vi "Plugin-002-CalibrationTest.vi"(0 "Configuration Page":refnum<class "Material-ConfigPage.lvclass">, 11 "error in":errorcluster) -> (15 "error out":errorcluster)   [LabVIEW 2014, in "Calibration-RunTest.lvclass"]
doc: "DisplayName=\"Deploy Configuration Template\"\nDescription=\"This VI serves as a template page for the Deploy Configuration UI.\""
uses:
  Plugins/Run Calibration Test/Calibration-RunTest.lvclass
  Reuse Library/featherweight/Core/Sequencer/FTW-Sequencer.lvclass
  Reuse Library/featherweight/Core/Messaging/Message.Actor/FTW-Message-Actor.lvclass
  Material-ConfigPage.lvclass
  <vilib>/Utility/miscctls.llb/LVPointTypeDef.ctl
  Plugins/Motion Control/Motion-ControlAll.lvclass
  Reuse Library/Keyence LK-G5000/Keyence LK-G5000.lvlib
  Reuse Library/Keyence LK-G5000/Public/Constant/Comm Interface.ctl
  <vilib>/Utility/error.llb/Error Cluster From Error Code.vi
  <vilib>/ErrorRing/Error Ring.xnode
panel:
  out "Thickness Measured Real Time":dbl format="%_6g"
  in  "Stop Button":bool
  out "Calibration Complete":bool
  in  "Collect Cal Data":bool
  out "Line 3 Calibration Data":dbl[](graph)
  out "Line 2 Calibration Data":dbl[](graph)
  out "Line 1 Calibration Data":dbl[](graph)
  # "Inputs"
  # "Outputs"
  # "Second Plugin"
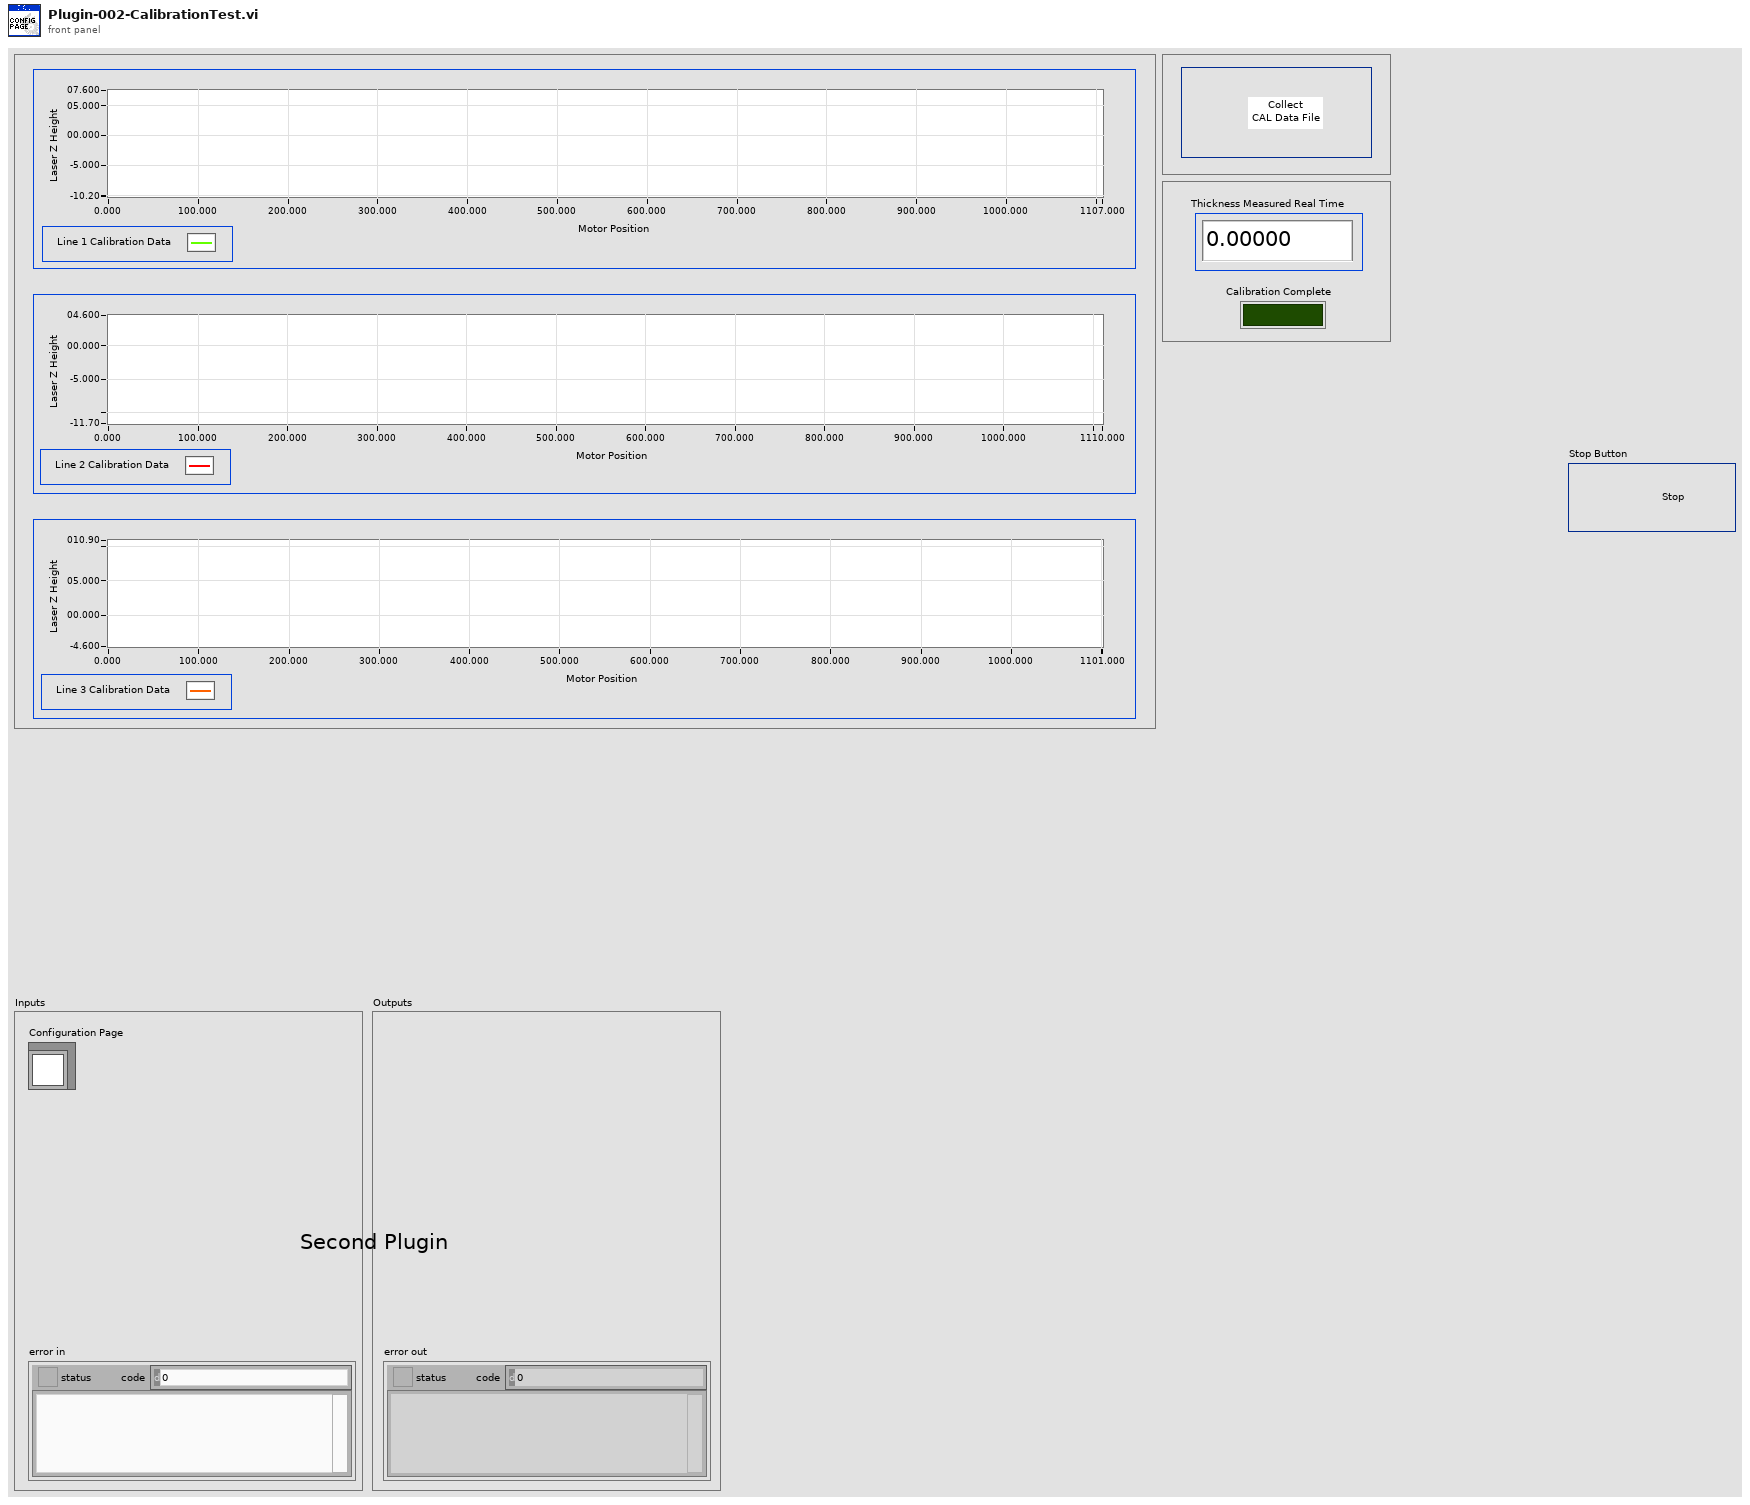
[diagram p1: front panel]
types:
  T1 = enum8{"Enabled", "Disabled", "Disabled and Grayed Out"}
  T2 = typedef "Keyence LK-G5000.lvlib/Comm Interface.ctl" = enum8{"USB", "ETHERNET"}
  T3 = typedef "LVPointTypeDef.ctl" = cluster{"Horizontal":i16, "Vertical":i16}
  T4 = cluster{"PageCommands":refnum<event-registration>}
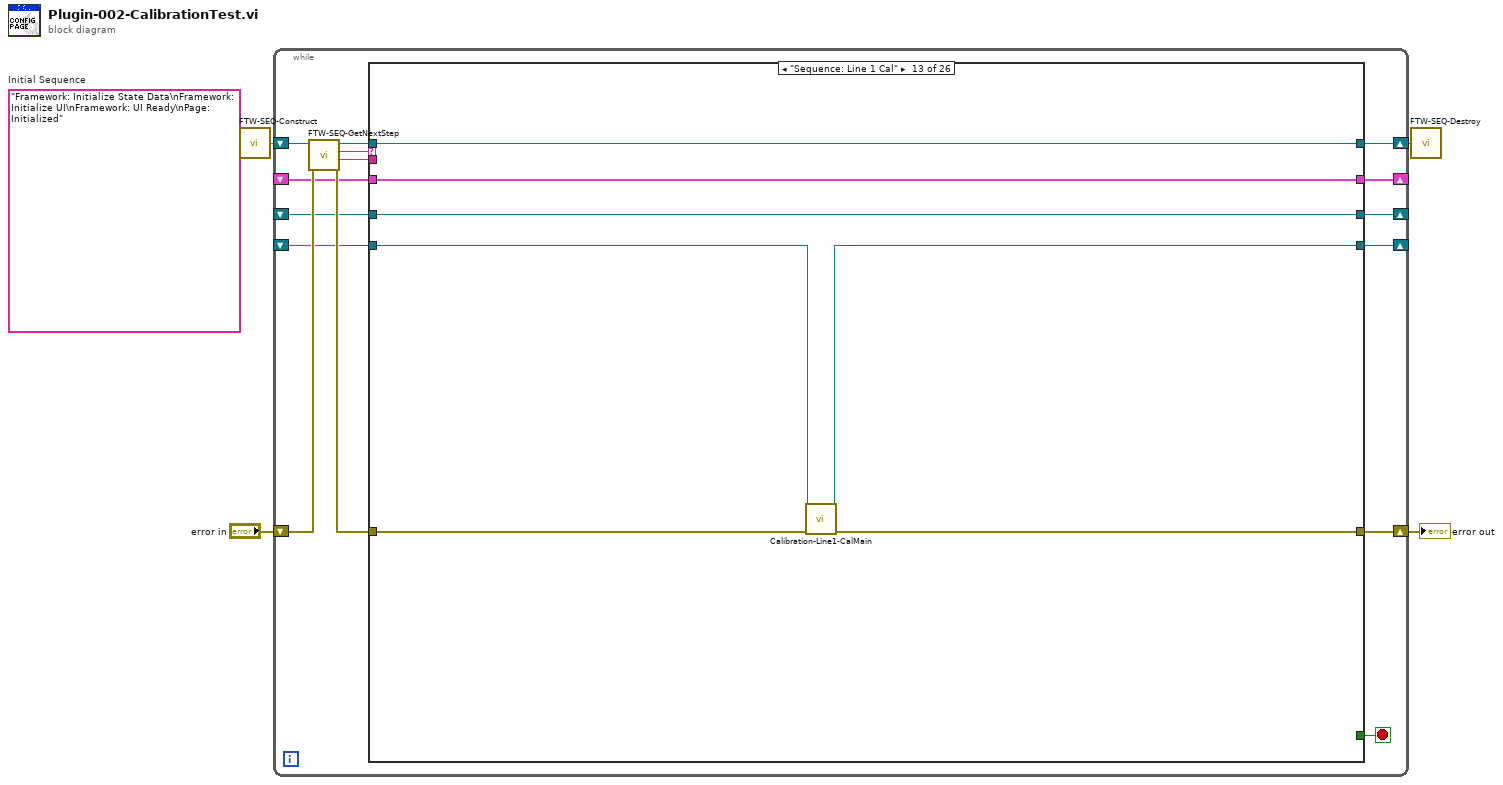
[diagram p0: block diagram]
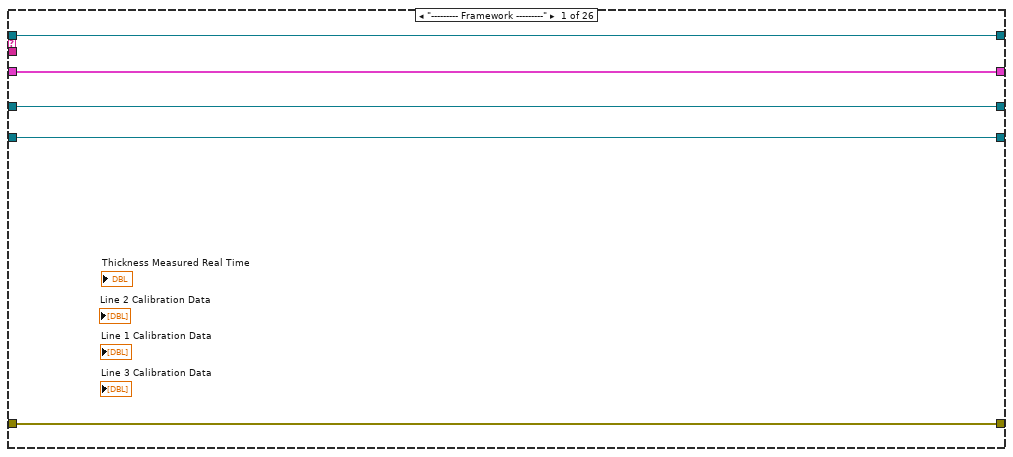
[diagram p2: hidden frame]
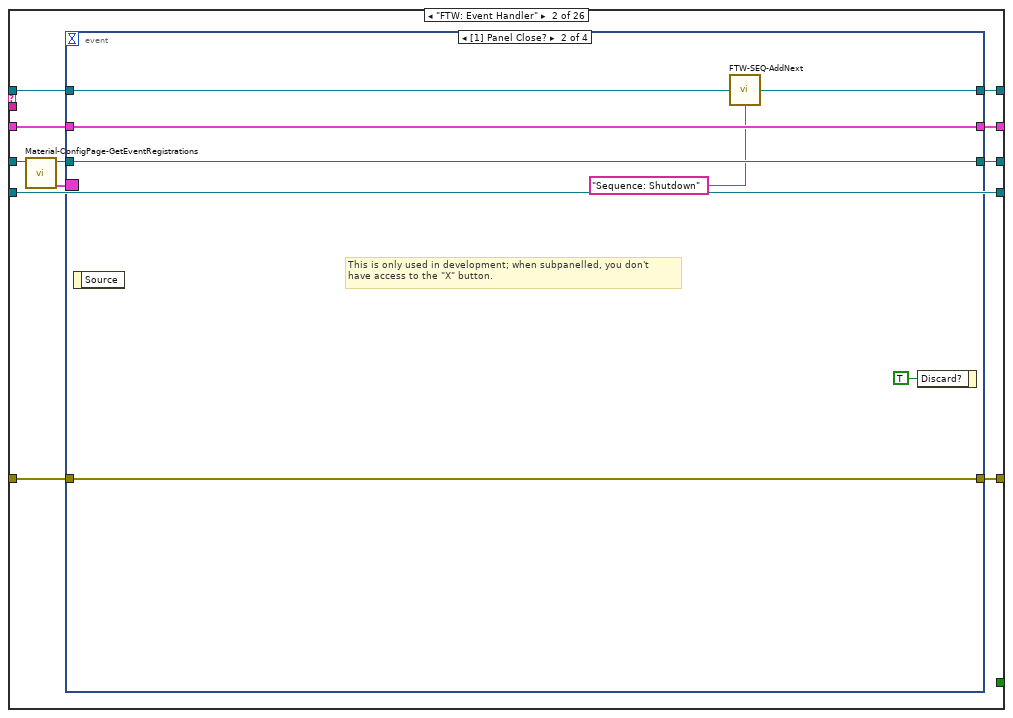
[diagram p3: hidden frame]
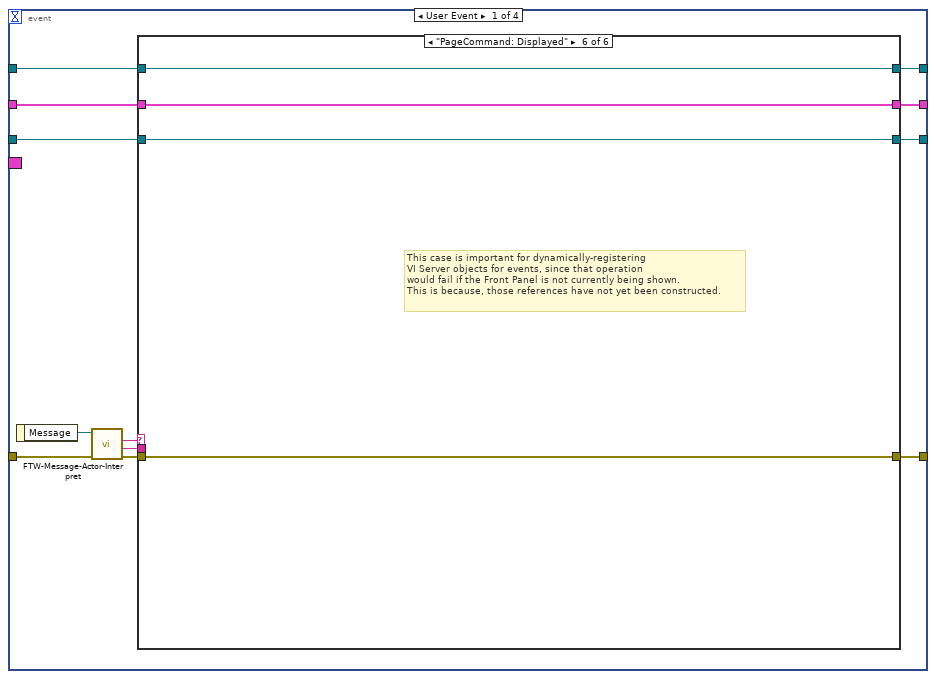
[diagram p4: hidden frame]
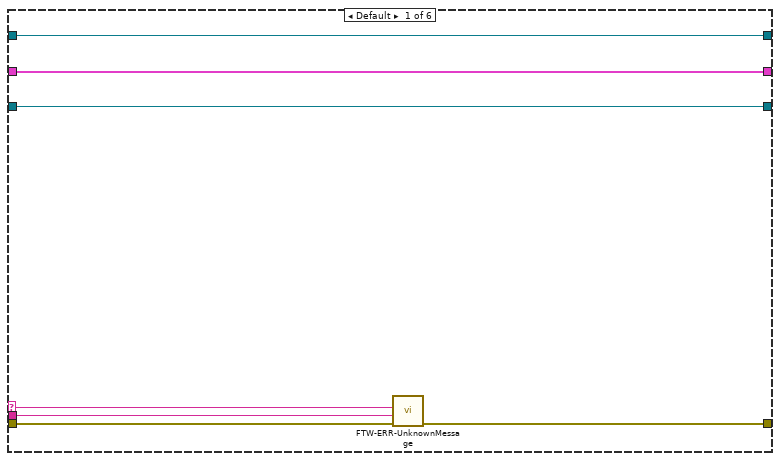
[diagram p5: hidden frame]
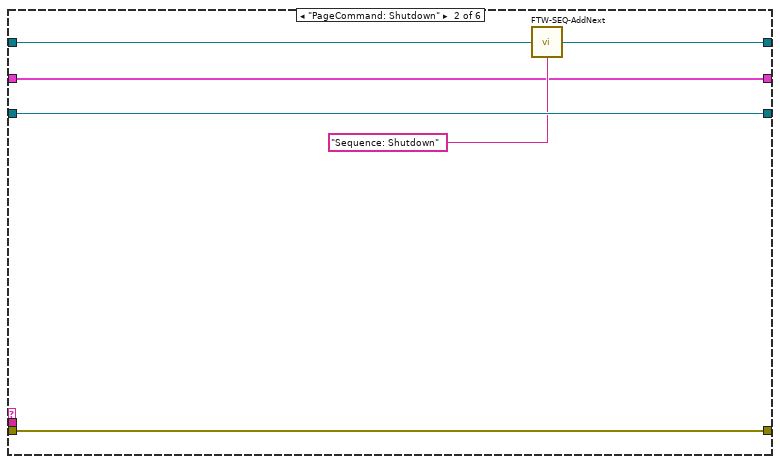
[diagram p6: hidden frame]
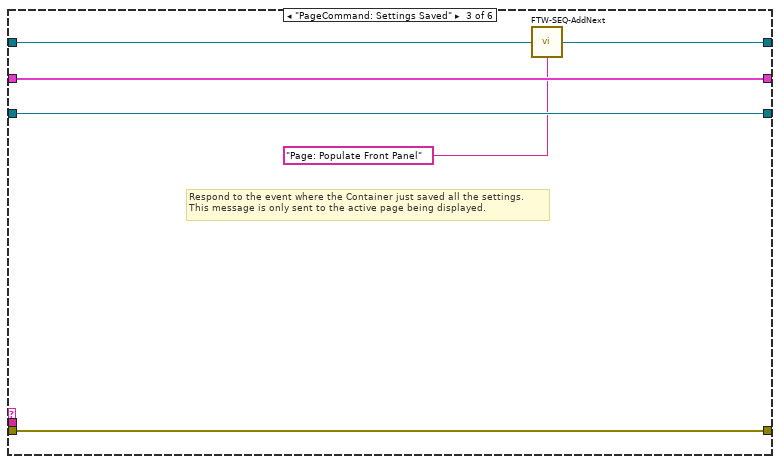
[diagram p7: hidden frame]
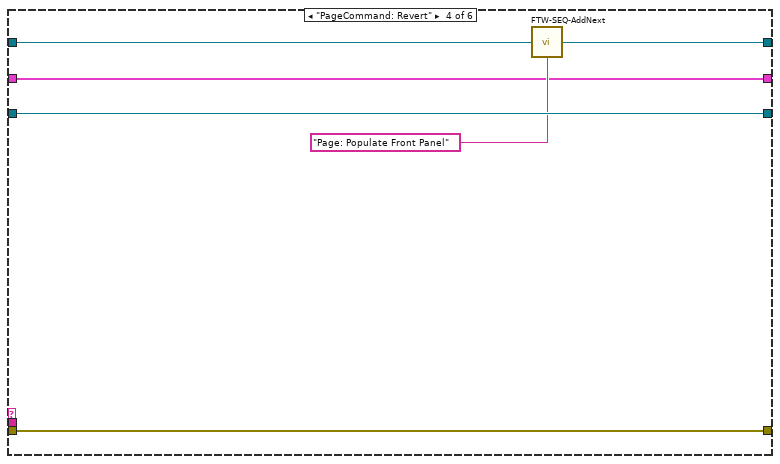
[diagram p8: hidden frame]
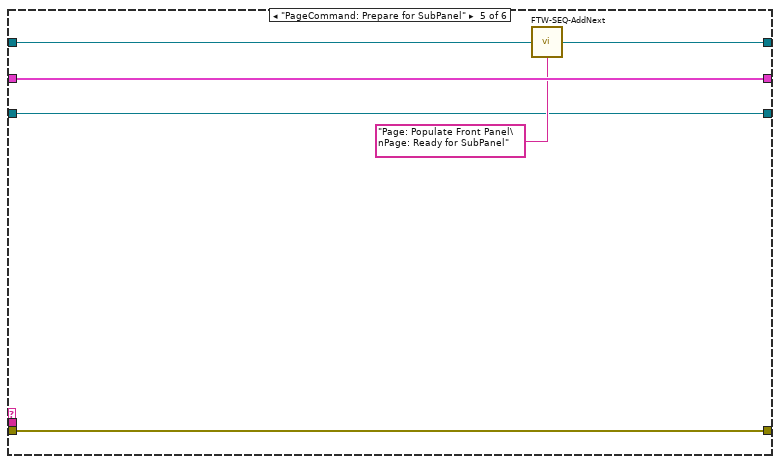
[diagram p9: hidden frame]
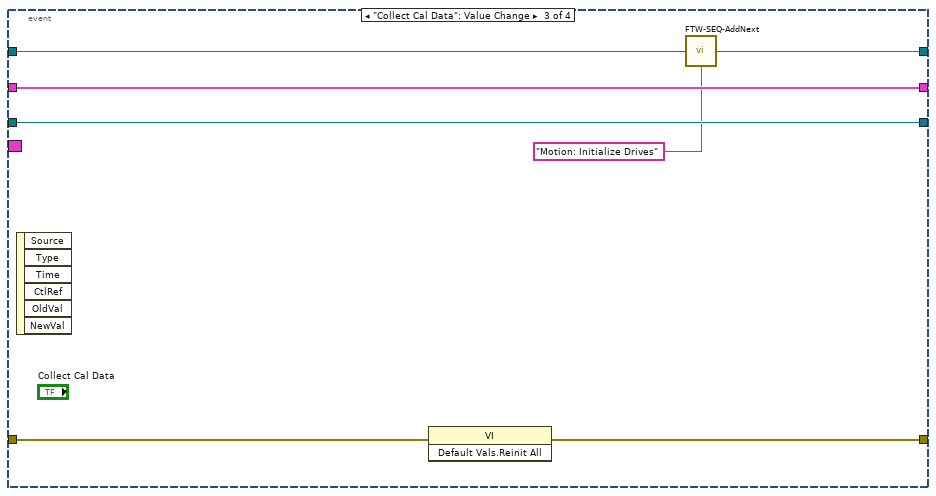
[diagram p10: hidden frame]
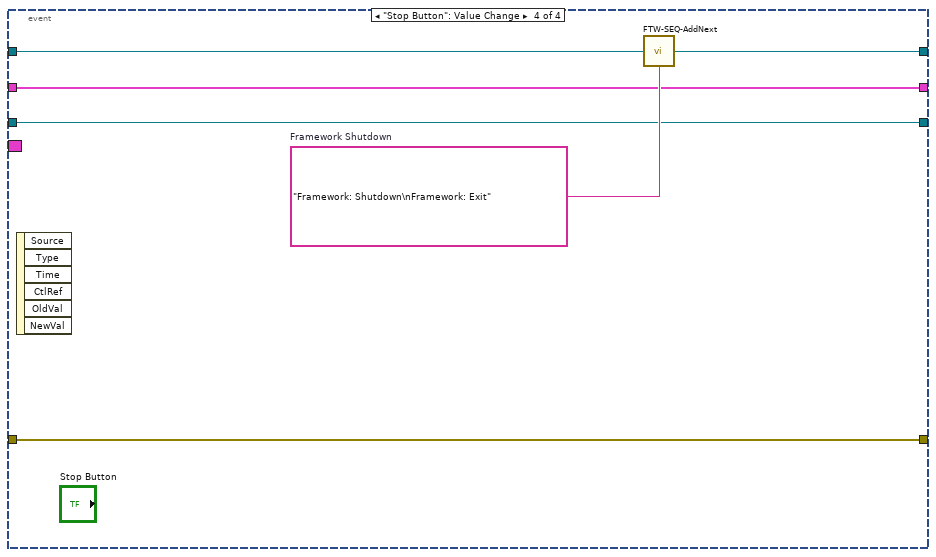
[diagram p11: hidden frame]
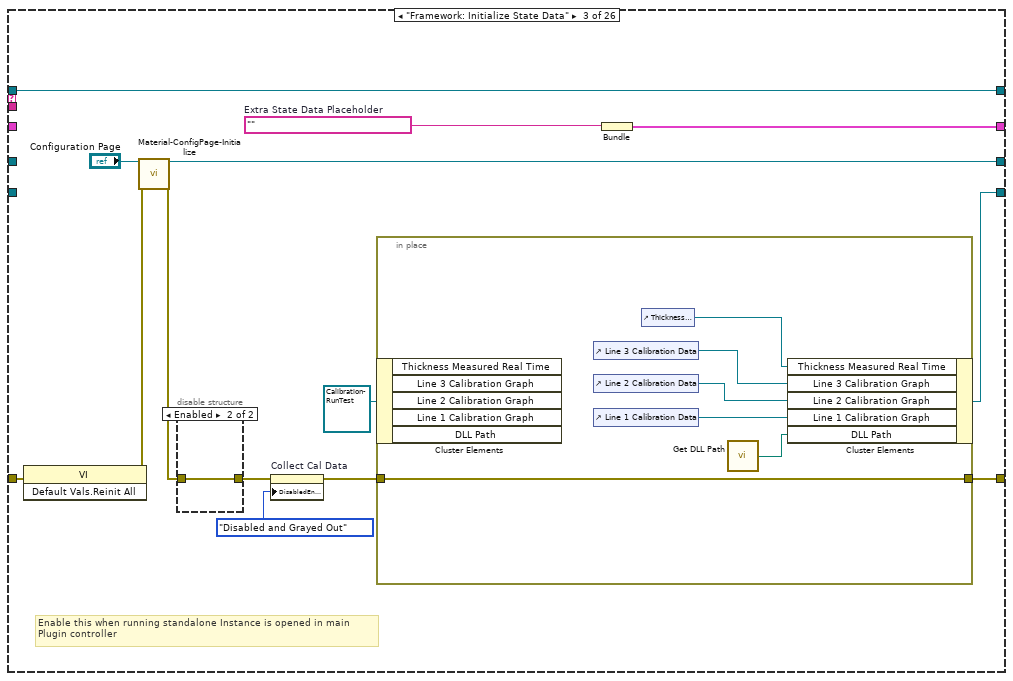
[diagram p12: hidden frame]
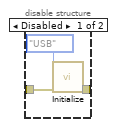
[diagram p13: hidden frame]
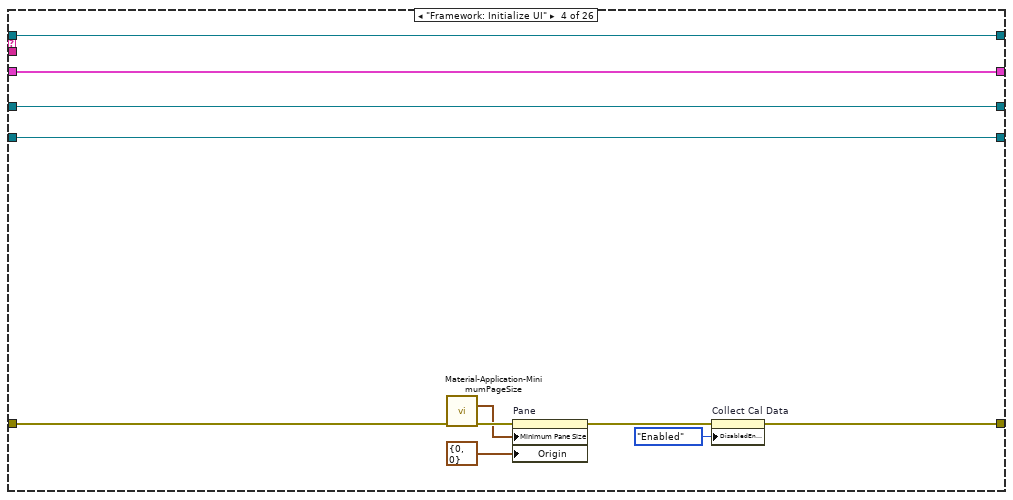
[diagram p14: hidden frame]
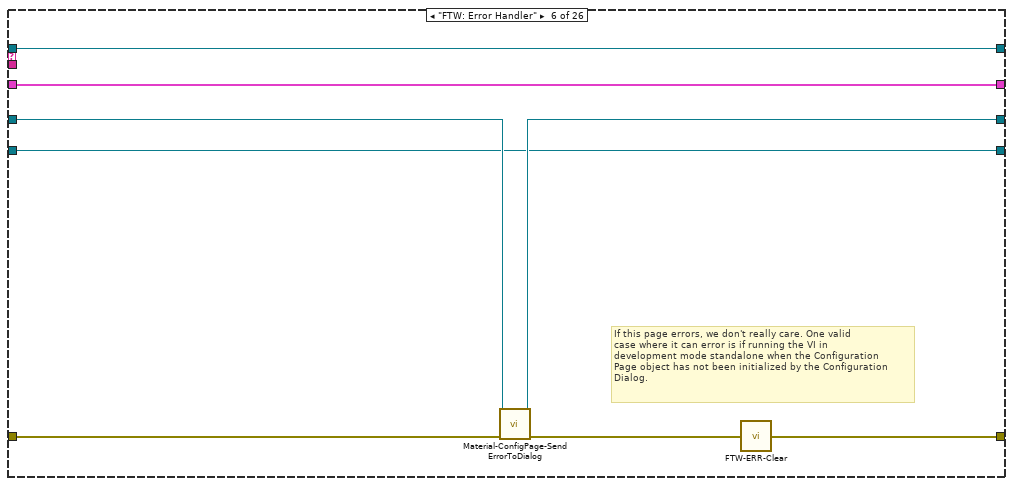
[diagram p16: hidden frame]
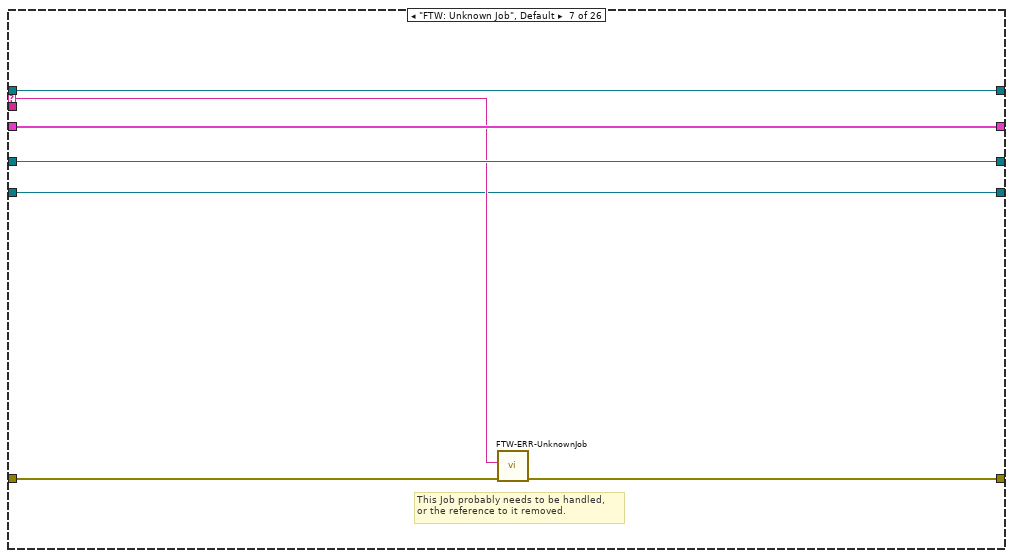
[diagram p17: hidden frame]
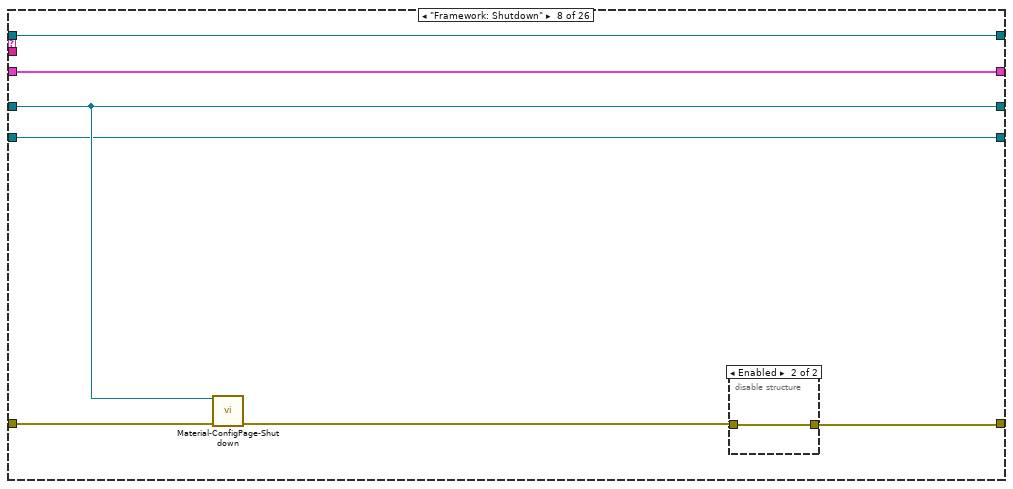
[diagram p18: hidden frame]
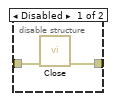
[diagram p19: hidden frame]
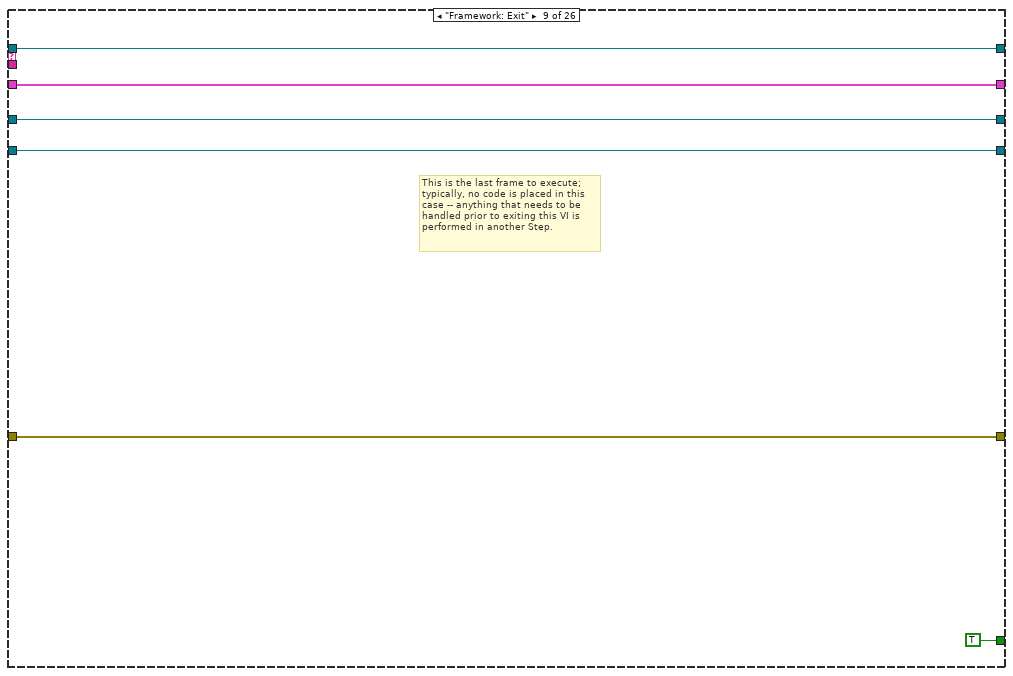
[diagram p20: hidden frame]
diagram:
  w5 = "Framework: Initialize State Data\nFramework: Initialize UI\nFramework: UI Ready\nPage: Initialized"  # Initial Sequence
  n1 = call "FTW-SEQ-Construct.vi"("Initial Sequence"=w5) -> ("Sequencer"=w4:refnum<class "FTW-Sequencer.lvclass">)
  n2 = while {
    shift-right: [w18] -> w3
    shift-left: w4 -> [w9]
    shift-right: [w19] -> w2
    shift-left: "error in" -> [w17]
    shift-right: [w13] -> _
    shift-left: _ -> [w12]
    shift-right: [w11] -> _
    shift-left: _ -> [w10]
    shift-right: [w7] -> _
    shift-left: _ -> [w6]
    stop <- w14 stop-if-true
    n3 = call "FTW-SEQ-GetNextStep.vi"("error in"=w17, "Sequencer"=w9) -> ("error out"=w20:errorcluster, "Job Data"=w8:string, "Current Job"=w15:string, "Sequencer out"=w16:refnum<class "FTW-Sequencer.lvclass">)  [unwired: 6 in]
    n4 = case shown="\"Sequence: Line 1 Cal\"" w15 {
      selector: w15 -> [_ _ _ _ _ _ w153 _ _ _ _ _ _ _ _ _ _ _ _ _ _ _ _ _ _ _]
      tunnel: [w23 w34 w109 w128 w143 w150 w155 w161 w172 w180 w187 w192 w209 w216 w223 w234 w244 w252 w258 w262 w271 w273 w282 w307 w319 w330] -> w19
      tunnel: w20 -> [w23 w33 w112 w134 w143 w147 w156 w163 w172 w180 w187 w193 w212 w219 w226 w231 w245 w252 w259 w262 w272 w273 w288 w310 w320 w331]
      tunnel: w16 -> [w24 w36 w116 w133 w140 w145 w158 w164 w170 w177 w184 w189 w215 w222 w229 w237 w240 w249 w255 w265 w267 w276 w279 w306 w322 w333]
      tunnel: [w24 w35 w116 w133 w140 w145 w158 w164 w170 w176 w183 w189 w215 w222 w229 w237 w239 w249 w255 w265 w267 w276 w281 w305 w322 w333] -> w18
      tunnel: [_ _ _ _ _ _ _ _ TRUE _ _ _ _ _ _ _ _ _ _ _ _ _ _ _ _ _] -> w14
      tunnel: [w25 w32 w117 w138 w142 w151 w157 w165 w173 w181 w188 w195 w214 w221 w228 w236 w247 w251 w260 w264 w270 w277 w290 w312 w323 w334] -> w13
      tunnel: w12 -> [w25 w30 _ w138 w142 w151 w157 w165 w173 w181 w188 w195 w214 w221 w228 w236 w247 w251 w260 w264 w270 w277 w290 w312 w323 w334]
      tunnel: [w22 w31 w115 w137 w141 w148 w154 w162 w171 w179 w186 w194 w213 w220 w227 w235 w246 w250 w256 w263 w268 w274 w289 w311 w321 w332] -> w11
      tunnel: w10 -> [w22 w29 _ w137 w141 w149 w154 w162 w171 w179 w186 w194 w213 w220 w227 w235 w246 w250 w257 w263 w269 w274 w289 w311 w321 w332]
      tunnel: w8 -> [_ _ _ _ _ _ _ _ _ _ _ _ _ _ _ _ _ _ _ _ _ _ _ _ _ _]
      tunnel: [w21 w26 w108 w131 w139 w144 w152 w159 w169 w175 w182 w190 w210 w217 w224 w232 w242 w248 w253 w261 w266 w275 w278 w308 w317 w328] -> w7
      tunnel: w6 -> [w21 w26 _ w131 w139 w144 w152 w159 w169 w175 w182 w191 w211 w218 w225 w233 w243 w248 w253 w261 w266 w275 w287 w309 w318 w329]
      frame "--------- Framework ---------" {
      }
      frame "FTW: Event Handler" {
        n5 = call "Material-ConfigPage-GetEventRegistrations.vi"("Configuration Page"=w29) -> ("Events"=w27:T4, "Configuration Page out"=w28:refnum<class "Material-ConfigPage.lvclass">)  [unwired: 9 in]
        n6 = event shown="[1] Panel Close?" {
          selector: w27 -> [_ _ _ _]
          dyn-events: _ -> [_ _ _ _]
          timeout: _ -> [_ _ _ _]
          tunnel: w36 -> [w42 w85 w93 w102]
          tunnel: [w43 w84 w94 w103] -> w35
          tunnel: [w47 w88 w91 w98] -> w34
          tunnel: w33 -> [w48 w88 w92 w98]
          tunnel: [w41 w89 w96 w100] -> w32
          tunnel: w30 -> [w40 w89 w96 w100]
          tunnel: w28 -> [w45 w87 w97 w99]
          tunnel: [w44 w87 w97 w99] -> w31
          event User Event {
            n7 = event-data() -> ("Message"=w38:refnum<class "FTW-Message.lvclass">)  [unwired: 1 in]
            n8 = call "FTW-Message-Actor-Interpret.vi"("error in"=w48, "Message"=w38) -> ("error out"=w46:errorcluster, "Sender"=w37:string, "Parameter"=w39:string)  [unwired: 6 in, 1 out]
            n9 = case shown="\"PageCommand: Displayed\"" w39 {
              selector: w39 -> [w50 _ _ _ _ _]
              tunnel: [w54 w61 w67 w73 w74 w80] -> w47
              tunnel: w46 -> [w55 w61 w67 w73 w74 w80]
              tunnel: w45 -> [w53 w60 w66 w72 w75 w81]
              tunnel: [w53 w60 w66 w72 w75 w81] -> w44
              tunnel: [w52 w56 w64 w70 w78 w82] -> w43
              tunnel: w42 -> [w52 w59 w65 w71 w79 w82]
              tunnel: [w51 w57 w63 w68 w77 w83] -> w41
              tunnel: w40 -> [w51 w57 w63 w68 w77 w83]
              tunnel: w37 -> [w49 _ _ _ _ _]
              frame Default {
                n10 = call "FTW-ERR-UnknownMessage.vi"("error in"=w55, "Sender"=w49, "Unknown Parameter"=w50) -> ("error out"=w54:errorcluster)  [unwired: 8 in]
              }
              frame "PageCommand: Shutdown" {
                n11 = call "FTW-SEQ-AddNext.vi"("Add Next in Sequence"="Sequence: Shutdown", "Sequencer"=w59) -> ("Sequencer out"=w56:refnum<class "FTW-Sequencer.lvclass">)  [unwired: 2 in]
              }
              frame "PageCommand: Settings Saved" {
                # "Respond to the event where the Container just saved all the settings.\nThis message is only sent to the active page being displayed."
                n12 = call "FTW-SEQ-AddNext.vi"("Add Next in Sequence"="Page: Populate Front Panel" ("Add to Top of Sequence"), "Sequencer"=w65) -> ("Sequencer out"=w64:refnum<class "FTW-Sequencer.lvclass">)  [unwired: 2 in]
              }
              frame "PageCommand: Revert" {
                n13 = call "FTW-SEQ-AddNext.vi"("Add Next in Sequence"="Page: Populate Front Panel", "Sequencer"=w71) -> ("Sequencer out"=w70:refnum<class "FTW-Sequencer.lvclass">)  [unwired: 2 in]
              }
              frame "PageCommand: Prepare for SubPanel" {
                n14 = call "FTW-SEQ-AddNext.vi"("Add Next in Sequence"="Page: Populate Front Panel\nPage: Ready for SubPanel", "Sequencer"=w79) -> ("Sequencer out"=w78:refnum<class "FTW-Sequencer.lvclass">)  [unwired: 2 in]
              }
              frame "PageCommand: Displayed" {
                # "This case is important for dynamically-registering\nVI Server objects for events, since that operation\nwould fail if the Front Panel is not currently being shown.\nThis is because, those references have not yet been constructed."
              }
            }
          }
          event Panel Close? {
            # "This is only used in development; when subpanelled, you don't\nhave access to the \"X\" button."
            n15 = event-data() -> ()  [unwired: 1 in, 1 out]
            n16 = call "FTW-SEQ-AddNext.vi"("Add Next in Sequence"="Sequence: Shutdown" ("Add to Top of Queue"), "Sequencer"=w85) -> ("Sequencer out"=w84:refnum<class "FTW-Sequencer.lvclass">)  [unwired: 2 in]
            n17 = event-data("Discard?"=TRUE) -> ()  [unwired: 1 in, 1 out]
          }
          event "Collect Cal Data": Value Change {
            n18 = event-data() -> ()  [unwired: 1 in, 6 out]
            n19 = invoke class="VI" method="Default Vals.Reinit All"(error in=w92) -> (error out=w91:errorcluster)  [unwired: 2 in, 2 out]
            n20 = call "FTW-SEQ-AddNext.vi"("Add Next in Sequence"="Motion: Initialize Drives" ("Add to Top of Queue"), "Sequencer"=w93) -> ("Sequencer out"=w94:refnum<class "FTW-Sequencer.lvclass">)  [unwired: 2 in]
          }
          event "Stop Button": Value Change {
            w101 = "Framework: Shutdown\nFramework: Exit"  # Framework Shutdown
            n21 = event-data() -> ()  [unwired: 1 in, 6 out]
            n22 = call "FTW-SEQ-AddNext.vi"("Add Next in Sequence"=w101, "Sequencer"=w102) -> ("Sequencer out"=w103:refnum<class "FTW-Sequencer.lvclass">)  [unwired: 2 in]
          }
        }
      }
      frame "Framework: Initialize State Data" {
        w114 = ""  # Extra State Data Placeholder
        # "Enable this when running standalone Instance is opened in main\nPlugin controller"
        n23 = invoke class="VI" method="Default Vals.Reinit All"(error in=w112) -> (error out=w111:errorcluster)  [unwired: 2 in, 2 out]
        n24 = call-dynamic "Material-ConfigPage-Initialize.vi"("Configuration Page"="Configuration Page", "error in"=w111) -> ("Configuration Page out"=w115:refnum<class "Material-ConfigPage.lvclass">, "error out"=w104:errorcluster)  [unwired: 12 in]
        n25 = disable-structure shown="Enabled" {
          disable-tunnel: w104 -> [w125 w127]
          disable-tunnel: [w124 w127] -> w106
          frame Disabled {
            n26 = call "Initialize.vi"("error in (no error)"=w125, "Comm Interface"=Comm_Interface."USB") -> ("error out"=w124:errorcluster)  [unwired: 9 in]
          }
          frame Enabled {
          }
        }
        n27 = property on="Collect Cal Data" class="Bool"(error in=w106, "DisabledEnum"=T1."Disabled and Grayed Out" ("Disabled")) -> (error out=w105:errorcluster)  [unwired: 1 in, 1 out]
        n28 = in-place {
          in-place-border: w105 -> [w119]
          in-place-border: [w119] -> w109
          n29 = in-place-cluster #1(refnum<class "Calibration-RunTest.lvclass"> refnum ("Calibration-RunTest.lvclass")) -> ()  [unwired: 5 out]
          n30 = control-ref of="Line 3 Calibration Data"() -> (w121:refnum<vi>)
          n31 = control-ref of="Line 2 Calibration Data"() -> (w122:refnum<vi>)
          n32 = control-ref of="Line 1 Calibration Data"() -> (w123:refnum<vi>)
          n33 = control-ref of="Thickness Measured Real Time"() -> (w120:refnum<vi>)
          n34 = call "Get DLL Path.vi"() -> ("DLL Path"=w118:path)  [unwired: 1 in]
          n35 = in-place-cluster #1("Thickness Measured Real Time"=w120, "Line 3 Calibration Graph"=w121, "Line 2 Calibration Graph"=w122, "Line 1 Calibration Graph"=w123, "DLL Path"=w118) -> (w108:refnum<class "Calibration-RunTest.lvclass">)
        }
        n36 = Bundle("Extra State Data Placeholder"=w114) -> (w117:cluster{"Extra State Data Placeholder":string})  [unwired: 1 in]
      }
      frame "Framework: Initialize UI" {
        n37 = call "Material-Application-MinimumPageSize.vi"("error in"=w134) -> ("Minimum Pane Size"=w135:cluster{"Horizontal":i16, "Vertical":i16}, "error out"=w136:errorcluster)  [unwired: 13 in]
        n38 = property on="Pane" class="Pane"(error in=w136, "Minimum Pane Size"=w135, "Origin"=T3 {"Horizontal"=0, "Vertical"=0}) -> (error out=w130:errorcluster)  [unwired: 1 in, 1 out]
        n39 = property on="Collect Cal Data" class="Bool"(error in=w130, "DisabledEnum"=T1."Enabled" ("Disabled")) -> (error out=w128:errorcluster)  [unwired: 1 in, 1 out]
      }
      frame "Framework: UI Ready" {
      }
      frame "FTW: Error Handler" {
        # "If this page errors, we don't really care. One valid\ncase where it can error is if running the VI in\ndevelopment mode standalone when the Configuration\nPage object has not been initialized by the Configuration\nDialog."
        n40 = call "Material-ConfigPage-SendErrorToDialog.vi"("Configuration Page in"=w149, "error in"=w147) -> ("Configuration Page out"=w148:refnum<class "Material-ConfigPage.lvclass">, "error out"=w146:errorcluster)  [unwired: 12 in]
        n41 = call "FTW-ERR-Clear.vi"("error to snuff"=w146) -> ("no error"=w150:errorcluster)
      }
      frame "FTW: Unknown Job", Default {
        # "This Job probably needs to be handled,\nor the reference to it removed."
        n42 = call "FTW-ERR-UnknownJob.vi"("error in"=w156, "Unknown Job"=w153) -> ("error out"=w155:errorcluster)  [unwired: 9 in]
      }
      frame "Framework: Shutdown" {
        n43 = call "Material-ConfigPage-Shutdown.vi"("Configuration Page"=w162, "error in"=w163) -> ("error out"=w160:errorcluster)  [unwired: 13 in]
        n44 = disable-structure shown="Enabled" {
          disable-tunnel: w160 -> [w167 w168]
          disable-tunnel: [w166 w168] -> w161
          frame Disabled {
            n45 = call "Close.vi"("error in (no error)"=w167) -> ("error out"=w166:errorcluster)  [unwired: 10 in]
          }
          frame Enabled {
          }
        }
      }
      frame "Framework: Exit" {
        # "This is the last frame to execute;\ntypically, no code is placed in this\ncase -- anything that needs to be\nhandled prior to exiting this VI is\nperformed in another Step."
      }
      frame "--------- Sequences ---------" {
        w178 = ""  # Add to Top of Sequence
        n46 = call "FTW-SEQ-AddNext.vi"("Add Next in Sequence"=w178, "Sequencer"=w177) -> ("Sequencer out"=w176:refnum<class "FTW-Sequencer.lvclass">)  [unwired: 2 in]
      }
      frame "Sequence: Shutdown" {
        w185 = "Framework: Shutdown\nFramework: Exit"  # Framework Shutdown
        n47 = call "FTW-SEQ-AddNext.vi"("Add Next in Sequence"=w185, "Sequencer"=w184) -> ("Sequencer out"=w183:refnum<class "FTW-Sequencer.lvclass">)  [unwired: 2 in]
      }
      frame "Sequence: Zero Laser" {
        # "Steps: Move XY to Zero Position then perform and laser\nzeroing."
        n48 = in-place {
          in-place-border: w193 -> [w206]
          in-place-border: [w202] -> w192
          w198 = "MA1: A 10: V 20: AD 10: D " ("concatenated string")
          n49 = in-place-cluster #2(w191) -> ("Motion-ControlAll.lvclass"=w197:refnum<class "Motion-ControlAll.lvclass">)
          n50 = call "Motion-Move-XandY.vi"("Y Drive Acc/Speed/Velocity"=w198, "X Drive Acc/Speed/Velocity"=w198, "error in (no error)"=w206, "X Coordinates"="0", "Y Coordinates"="200000", "Motion-ControlAll in"=w197) -> ("error out"=w204:errorcluster, "Motion-ControlAll out"=w205:refnum<class "Motion-ControlAll.lvclass">)  [unwired: 4 in]
          n51 = call "Motion-PollAxis-Main.vi"("error in (no error)"=w204, "Motion-ControlAll in"=w205) -> ("error out"=w201:errorcluster, "Motion-ControlAll out"=w196:refnum<class "Motion-ControlAll.lvclass">)  [unwired: 8 in]
          n52 = call <vilib>:"Wait n mSec.vi"("error in (no error)"=w201, "Milliseconds to Wait (500)"=u32 1000) -> ("error out"=w199:errorcluster)  [unwired: 13 in]
          n53 = in-place-cluster #2("Motion-ControlAll.lvclass"=w196) -> (w190:refnum<class "Calibration-RunTest.lvclass">)
          n54 = call "LKIF2_SetZero.vi"("error in (no error)"=w199, "OnOff"=TRUE) -> ("error out"=w202:errorcluster)  [unwired: 9 in]
        }
      }
      frame "Sequence: Line 1 Cal" {
        n55 = call "Calibration-Line1-CalMain.vi"("error in (no error)"=w212, "Calibration-RunTest in"=w211) -> ("error out"=w209:errorcluster, "Calibration-RunTest out"=w210:refnum<class "Calibration-RunTest.lvclass">)  [unwired: 8 in]
      }
      frame "Sequence: Line 2 Cal" {
        n56 = call "Calibration-Line2-CalMain.vi"("error in (no error)"=w219, "Calibration-RunTest in"=w218) -> ("error out"=w216:errorcluster, "Calibration-RunTest out"=w217:refnum<class "Calibration-RunTest.lvclass">)  [unwired: 8 in]
      }
      frame "Sequence: Line 3 Cal" {
        n57 = call "Calibration-Line3-CalMain.vi"("error in (no error)"=w226, "Calibration-RunTest in"=w225) -> ("error out"=w223:errorcluster, "Calibration-RunTest out"=w224:refnum<class "Calibration-RunTest.lvclass">)  [unwired: 8 in]
      }
      frame "Sequence: Normalize Data" {
        n58 = call "Calibration-Splash-Normalizing.vi"("error in (no error)"=w231) -> ("error out"=w230:errorcluster)  [unwired: 10 in]
        n59 = call "Calibration-NormalizeData.vi"("error in (no error)"=w230, "Calibration-RunTest in"=w233) -> ("error out"=w234:errorcluster, "Calibration-RunTest out"=w232:refnum<class "Calibration-RunTest.lvclass">)  [unwired: 8 in]
      }
      frame "Sequence: Save Data?" {
        n60 = call "Calibration-SaveData.vi"("error in (no error)"=w245, "Calibration-RunTest in"=w243) -> ("error out"=w244:errorcluster, "Cal Finished"=→"Calibration Complete":bool, "Calibration-RunTest out"=w242:refnum<class "Calibration-RunTest.lvclass">)  [unwired: 7 in]
        n61 = call "FTW-SEQ-AddNext.vi"("Add Next in Sequence"="Sequence: Zero Laser\nMotion: DeEnergize Drives\nMotion: Close Connection" ("Add to Top of Queue"), "Sequencer"=w240) -> ("Sequencer out"=w239:refnum<class "FTW-Sequencer.lvclass">)  [unwired: 2 in]
      }
      frame "--------- Application Logic ---------" {
      }
      frame "Page: Initialized" {
        w254 = TRUE  # Allow user to open Diagram from SubPanel?
        n62 = call "Material-ConfigPage-Initialized.vi"("Configuration Page"=w257, "Allow user to open Diagram from SubPanel?"=w254, "error in"=w259) -> ("Configuration Page out"=w256:refnum<class "Material-ConfigPage.lvclass">, "error out"=w258:errorcluster)  [unwired: 11 in]
      }
      frame "Page: Populate Front Panel" {
      }
      frame "Page: Ready for SubPanel" {
        n63 = call "Material-ConfigPage-ReadyForSubPanel.vi"("Configuration Page"=w269, "error in"=w272) -> ("Configuration Page out"=w268:refnum<class "Material-ConfigPage.lvclass">, "error out"=w271:errorcluster)  [unwired: 12 in]
      }
      frame "----------Motion Control------------" {
      }
      frame "Motion: Initialize Drives" {
        n64 = in-place {
          in-place-border: w288 -> [w303]
          in-place-border: [w300] -> w283
          n65 = in-place-cluster #3(w287) -> ("Motion-ControlAll.lvclass"=w302:refnum<class "Motion-ControlAll.lvclass">)
          n66 = call "Motion-Intialize-Drives.vi"("error in (no error)"=w303, "Motion-ControlAll in"=w302) -> ("error out"=w300:errorcluster, "Motion-ControlAll out"=w301:refnum<class "Motion-ControlAll.lvclass">)  [unwired: 8 in]
          n67 = in-place-cluster #3("Motion-ControlAll.lvclass"=w301) -> (w278:refnum<class "Calibration-RunTest.lvclass">)
        }
        n68 = Unbundle By Name(w283) -> ("status"=w284:bool)
        n69 = Equal?(x=TRUE, y=w284) -> (x = y?=w286:bool)
        n70 = case shown="False" w286 {
          tunnel: ["Motion: Energize Drives" ("Add to Top of Queue") "" ("Begin Test Sequence")] -> w280
          tunnel: w283 -> [w292 _]
          tunnel: [w292 w293] -> w282
          frame False {
          }
          frame True {
            n71 = xnode "Error Ring"() -> ("error out"=w293:errorcluster)
          }
        }
        n72 = call "FTW-SEQ-AddNext.vi"("Add Next in Sequence"=w280, "Sequencer"=w279) -> ("Sequencer out"=w281:refnum<class "FTW-Sequencer.lvclass">)  [unwired: 2 in]
      }
      frame "Motion: Energize Drives" {
        w304 = "Sequence: Zero Laser\nSequence: Line 1 Cal\nSequence: Line 2 Cal\nSequence: Line 3 Cal\nSequence: Normalize Data\nSequence: Save Data?\n"  # Sequence Steps
        n73 = in-place {
          in-place-border: w310 -> [w316]
          in-place-border: [w315] -> w307
          n74 = in-place-cluster #4(w309) -> ("Motion-ControlAll.lvclass"=w314:refnum<class "Motion-ControlAll.lvclass">)
          n75 = call "Motion-Energize-Drives.vi"("error in (no error)"=w316, "Motion-ControlAll in"=w314) -> ("error out"=w315:errorcluster, "Motion-ControlAll out"=w313:refnum<class "Motion-ControlAll.lvclass">)  [unwired: 8 in]
          n76 = in-place-cluster #4("Motion-ControlAll.lvclass"=w313) -> (w308:refnum<class "Calibration-RunTest.lvclass">)
        }
        n77 = call "FTW-SEQ-AddNext.vi"("Add Next in Sequence"=w304, "Sequencer"=w306) -> ("Sequencer out"=w305:refnum<class "FTW-Sequencer.lvclass">)  [unwired: 2 in]
      }
      frame "Motion: DeEnergize Drives" {
        n78 = in-place {
          in-place-border: w320 -> [w327]
          in-place-border: [w324] -> w319
          n79 = in-place-cluster #5(w318) -> ("Motion-ControlAll.lvclass"=w326:refnum<class "Motion-ControlAll.lvclass">)
          n80 = call "Motion-DeEnergize-Drives.vi"("error in (no error)"=w327, "Motion-ControlAll in"=w326) -> ("error out"=w324:errorcluster, "Motion-ControlAll out"=w325:refnum<class "Motion-ControlAll.lvclass">)  [unwired: 8 in]
          n81 = in-place-cluster #5("Motion-ControlAll.lvclass"=w325) -> (w317:refnum<class "Calibration-RunTest.lvclass">)
        }
      }
      frame "Motion: Close Connection" {
        n82 = in-place {
          in-place-border: w331 -> [w338]
          in-place-border: [w337] -> w330
          n83 = in-place-cluster #6(w329) -> ("Motion-ControlAll.lvclass"=w335:refnum<class "Motion-ControlAll.lvclass">)
          n84 = call "Motion-Close.vi"("error in (no error)"=w338, "Motion-ControlAll in"=w335) -> ("error out"=w337:errorcluster, "Motion-ControlAll out"=w336:refnum<class "Motion-ControlAll.lvclass">)  [unwired: 8 in]
          n85 = in-place-cluster #6("Motion-ControlAll.lvclass"=w336) -> (w328:refnum<class "Calibration-RunTest.lvclass">)
        }
      }
    }
  }
  "error out" <- w2
  n86 = call "FTW-SEQ-Destroy.vi"("Sequencer"=w3) -> ()  [unwired: 1 in]
